vi "Acquire Analyze Visualize - Part 1.vi"() -> ()   [LabVIEW 2019]
uses:
  <vilib>/DAQmx/read.llb/DAQmx Read (Analog DBL 1Chan 1Samp).vi
  <vilib>/DAQmx/miscellaneous.llb/DAQmx Fill In Error Info.vi
panel:
  out "Current Temperature (deg C)":dbl format="%#_2f"
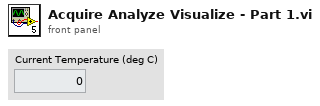
[diagram p1: front panel]
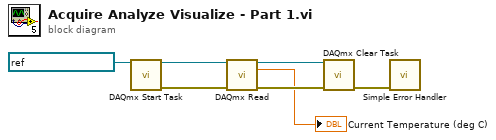
[diagram p0: block diagram]
diagram:
  n1 = call <vilib>:"DAQmx Start Task.vi"("task/channels in"=refnum<k21> "Thermocouple" ("DAQmx Task Name")) -> ("task out"=w4:refnum<k21>, "error out"=w6:errorcluster)  [unwired: 13 in]
  n2 = call-poly <vilib>:"DAQmx Read.vi"("task/channels in"=w4, "error in"=w6) -> ("task out"=w5:refnum<k21>, "data"=→"Current Temperature (deg C)":dbl, "error out"=w7:errorcluster)  [unwired: 11 in]
  n3 = call <vilib>:"DAQmx Clear Task.vi"("task in"=w5, "error in"=w7) -> ("error out"=w1:errorcluster)  [unwired: 13 in]
  n4 = call <vilib>:"Simple Error Handler.vi"("error in (no error)"=w1) -> ()  [unwired: 4 in, 5 out]
